vi "Write UDVs.vi"(7 "R/W Case":T4, 8 "error in (no error)":errorcluster, 9 "Input FIFO buffer in":dbl[](array[numeric]), 10 "Input Data in":T1 {"BD Refs"."Data Reference" format="%.0x"}, 11 "UDVs in":T5[](array[typedef]) {"VS ref" format="%.0x"}) -> (0 "error out":errorcluster, 1 "Input FIFO buffer out":dbl[](array[numeric]), 2 "Input Data out":T1 {"BD Refs"."Data Reference" format="%.0x"}, 3 "UDVs out":T5[](array[typedef]) {"VS ref" format="%.0x"})   [LabVIEW 2016, in "Scan Engine Custom Device.lvlib"]
uses:
  Scan Engine Custom Device.lvlib
  Type Defs/UDV Data.ctl
  <vilib>/NI Veristand/Custom Device API/Custom Device Item Ref.ctl
  Type Defs/UDV Data Type.ctl
  Type Defs/FXP Config.ctl
  Type Defs/RW Case.ctl
  Type Defs/Input Data.ctl
  <vilib>/NI Veristand/Custom Device API/Block Data Reference.ctl
  <vilib>/NI Veristand/Custom Device API/Data Reference.ctl
  <vilib>/NI Veristand/Custom Device API/Global Data Refs.vi
  <vilib>/NI Veristand/Custom Device API/Custom Device API.lvlib
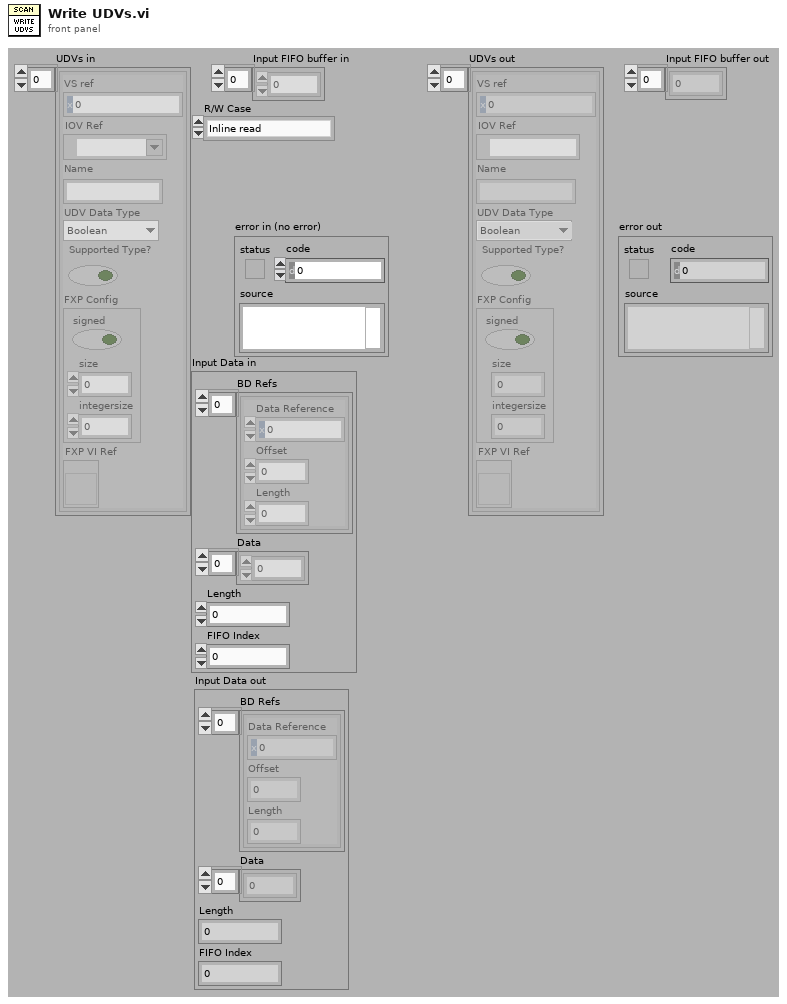
[diagram p1: front panel]
types:
  T1 = typedef "Scan Engine Custom Device.lvlib/Input Data.ctl" = cluster{"BD Refs":T2[], "Data":dbl[], "Length":i32, "FIFO Index":i32}
  T2 = typedef "Custom Device API.lvlib/Block Data Reference.ctl" = cluster{"Data Reference":T3, "Offset":u64, "Length":u64}
  T3 = typedef "Custom Device API.lvlib/Data Reference.ctl" = i32
  T4 = typedef "Scan Engine Custom Device.lvlib/RW Case.ctl" = enum16{"Inline read", "Inline write", "Async - Inline loop read", "Async - Inline loop write", "Async loop (read/write)"}
  T5 = typedef "Scan Engine Custom Device.lvlib/UDV Data.ctl" = cluster{"VS ref":T6, "IOV Ref":refnum<k21>, "Name":string, "UDV Data Type":T7, "Supported Type?":bool, "FXP Config":T8, "FXP VI Ref":refnum<vi>}
  T6 = typedef "Custom Device API.lvlib/Custom Device Item Ref.ctl" = u64
  T7 = typedef "Scan Engine Custom Device.lvlib/UDV Data Type.ctl" = enum16{"Boolean", "Fixed Point", "Int8", "Int16", "Int32", "Int64", "U32 Bit Field", "UInt8", "UInt16", "UInt32", "UInt64", "Other"}
  T8 = typedef "Scan Engine Custom Device.lvlib/FXP Config.ctl" = cluster{"signed":bool, "size":u32, "integersize":i32}
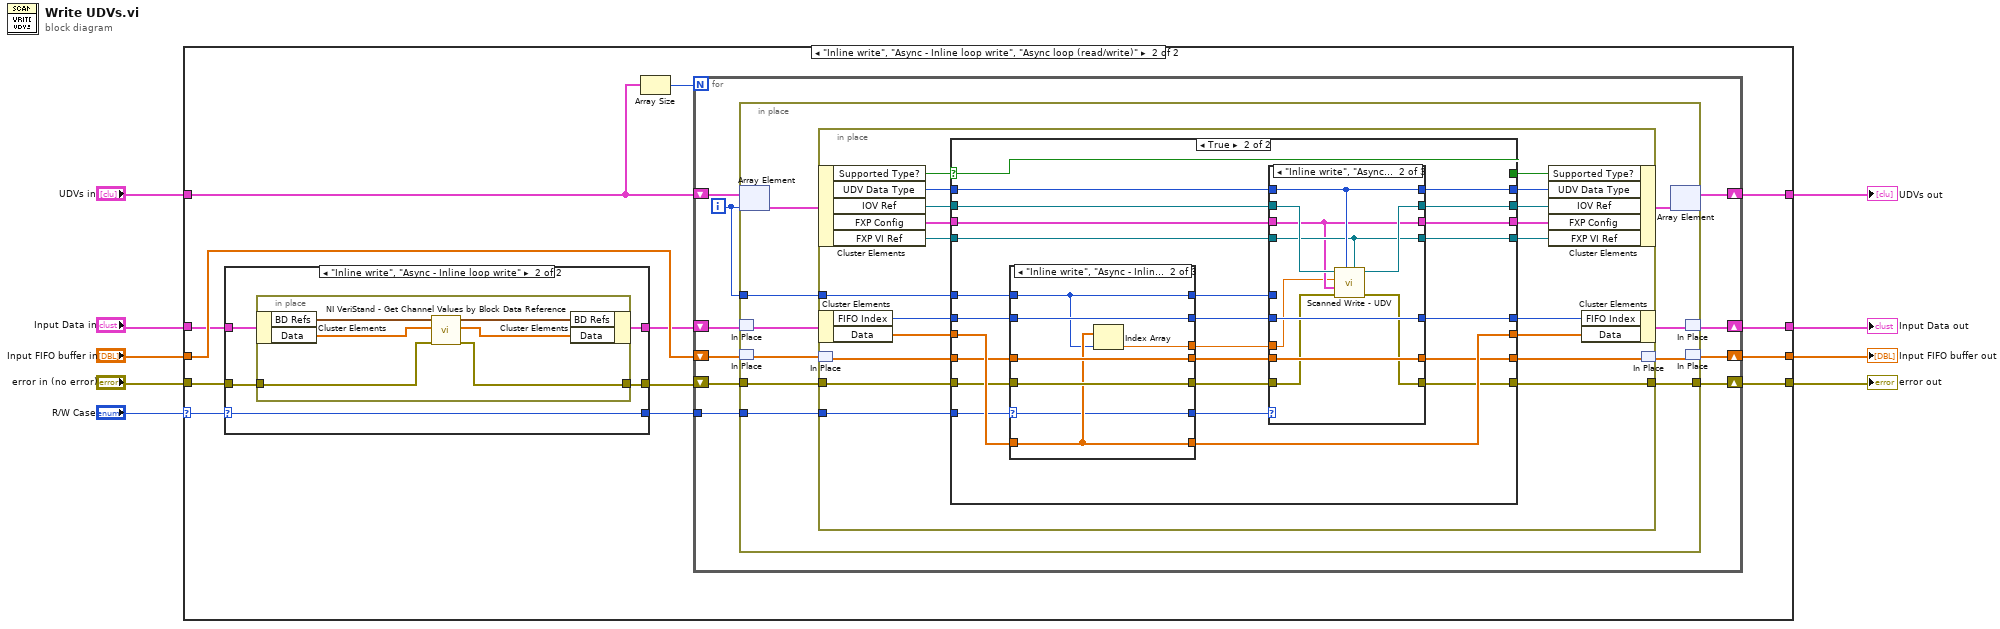
[diagram p0: block diagram]
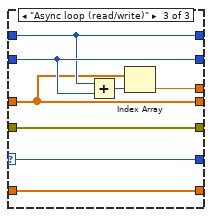
[diagram p6: hidden frame]
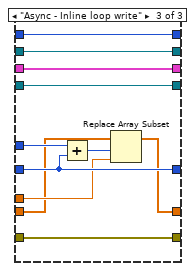
[diagram p8: hidden frame]
diagram:
  n1 = case shown="\"Inline write\", \"Async - Inline loop write\", \"Async loop (read/write)\"" "R/W Case" {
    selector: "R/W Case" -> [_ w21]
    tunnel: [w11 w26] -> w9
    tunnel: "Input FIFO buffer in" -> [w11 w25]
    tunnel: [w12 w15] -> w1
    tunnel: [w13 w24] -> w7
    tunnel: "Input Data in" -> [w12 w19]
    tunnel: "UDVs in" -> [w13 w23]
    tunnel: [w10 w14] -> w5
    tunnel: "error in (no error)" -> [w10 w20]
    frame Default {
    }
    frame "Inline write", "Async - Inline loop write", "Async loop (read/write)" {
      n2 = case shown="\"Inline write\", \"Async - Inline loop write\"" w21 {
        selector: w21 -> [w27 w30]
        tunnel: w19 -> [w28 w34]
        tunnel: w20 -> [w29 w33]
        tunnel: [w29 w32] -> w17
        tunnel: [w28 w31] -> w18
        tunnel: [w27 w30] -> w16
        frame Default {
        }
        frame "Inline write", "Async - Inline loop write" {
          n3 = in-place {
            in-place-border: w33 -> [w36]
            in-place-border: [w35] -> w32
            n4 = in-place-cluster #1(w34) -> ("BD Refs"=w40:T2[], "Data"=w38:dbl[])
            n5 = call <vilib>:"NI VeriStand - Get Channel Values by Block Data Reference.vi"("error in (no error)"=w36, "Values Array in"=w38, "Block Data Ref"=w40) -> ("error out"=w35:errorcluster, "Values Array out"=w37:dbl[], "Block Data Ref dup"=w39:T2[])  [unwired: 6 in]
            n6 = in-place-cluster #1("BD Refs"=w39, "Data"=w37) -> (w31:T1)
          }
        }
      }
      n7 = Array Size(array=w23) -> (size(s)=w22:i32)
      n8 = for {
        N: w22 -> [_]
        shift-right: [w49] -> w24
        shift-left: w23 -> [w50]
        shift-right: [w41] -> w15
        shift-left: w18 -> [w44]
        shift-right: [w47] -> w26
        shift-left: w25 -> [w48]
        shift-right: [w45] -> w14
        shift-left: w17 -> [w46]
        tunnel: w16 -> [w43]
        i -> [w42]
        n9 = in-place {
          in-place-border: w46 -> [w57]
          in-place-border: [w51] -> w45
          in-place-border: w43 -> [w56]
          in-place-border: w42 -> [w55]
          n10 = in-place-array #2(w50, w42) -> (w60:T5)
          n11 = in-place-match #3(w44) -> (w59:T1)
          n12 = in-place-match #4(w48) -> (w58:dbl[])
          n13 = in-place {
            in-place-border: w57 -> [w71]
            in-place-border: w56 -> [w61]
            in-place-border: w55 -> [w72]
            in-place-border: [w65] -> w51
            n14 = in-place-cluster #5(w60) -> ("Supported Type?"=w80:bool, "UDV Data Type"=w75:T7, "IOV Ref"=w74:refnum<k21>, "FXP Config"=w79:T8, "FXP VI Ref"=w78:refnum<vi>)
            n15 = in-place-cluster #6(w59) -> ("FIFO Index"=w77:i32, "Data"=w76:dbl[])
            n16 = in-place-match #7(w58) -> (w73:dbl[])
            n17 = case shown="True" w80 {
              selector: w80 -> [w88 w110]
              tunnel: w79 -> [w85 w112]
              tunnel: w78 -> [w84 w111]
              tunnel: w77 -> [w83 w100]
              tunnel: w76 -> [w82 w105]
              tunnel: w75 -> [w87 w114]
              tunnel: w74 -> [w86 w113]
              tunnel: w73 -> [w81 w99]
              tunnel: w72 -> [_ w101]
              tunnel: w71 -> [w89 w98]
              tunnel: [w88 w110] -> w70
              tunnel: [w87 w109] -> w69
              tunnel: [w86 w108] -> w68
              tunnel: [w85 w107] -> w67
              tunnel: [w84 w106] -> w66
              tunnel: [w89 w90] -> w65
              tunnel: [w83 w92] -> w64
              tunnel: [w82 w104] -> w63
              tunnel: [w81 w91] -> w62
              tunnel: w61 -> [_ w103]
              frame False {
              }
              frame True {
                n18 = case shown="\"Inline write\", \"Async - Inline loop write\"" w103 {
                  selector: w103 -> [w117 w121 w128]
                  tunnel: w101 -> [w115 w122 w130]
                  tunnel: w100 -> [w120 w125 w133]
                  tunnel: w99 -> [w118 w126 w129]
                  tunnel: w98 -> [w116 w127 w135]
                  tunnel: w105 -> [w119 w123 w134]
                  tunnel: [w120 w125 w133] -> w95
                  tunnel: [w119 w123 w134] -> w104
                  tunnel: [w116 w127 w135] -> w97
                  tunnel: [w118 w126 w129] -> w94
                  tunnel: [w117 w121 w128] -> w102
                  tunnel: [_ w124 w131] -> w93
                  tunnel: [w115 w122 w130] -> w96
                  frame Default {
                  }
                  frame "Inline write", "Async - Inline loop write" {
                    n19 = Index Array(array=w123, index=w122) -> (element=w124:dbl)
                  }
                  frame "Async loop (read/write)" {
                    n20 = Add(x=w130, y=w133) -> (x+y=w132:i32)
                    n21 = Index Array(array=w129, index=w132) -> (element=w131:dbl)
                  }
                }
                n22 = case shown="\"Inline write\", \"Async loop (read/write)\"" w102 {
                  tunnel: w114 -> [w136 w148 w161]
                  tunnel: w113 -> [w137 w150 w153]
                  tunnel: w112 -> [w138 w146 w163]
                  tunnel: w111 -> [w139 w147 w162]
                  tunnel: w95 -> [w140 w151 w158]
                  tunnel: w94 -> [w141 w152 w155]
                  tunnel: [w141 w152 w154] -> w91
                  tunnel: w96 -> [_ _ w159]
                  tunnel: [w140 w151 w158] -> w92
                  tunnel: [w137 w149 w153] -> w108
                  tunnel: [w136 w148 w161] -> w109
                  tunnel: [w138 w146 w163] -> w107
                  tunnel: [w139 w147 w162] -> w106
                  tunnel: w97 -> [w142 w144 w160]
                  tunnel: [w142 w143 w160] -> w90
                  tunnel: w93 -> [_ w145 w156]
                  frame Default {
                  }
                  frame "Inline write", "Async loop (read/write)" {
                    n23 = call "Scanned Write - UDV.vi"("FXP VI Ref"=w147, "UDV Data Type"=w148, "error in (no error)"=w144, "FXP Config"=w146, "data in"=w145, "IOV ref in"=w150) -> ("error out"=w143:errorcluster, "IOV ref out"=w149:refnum<k21>)  [unwired: 4 in]
                  }
                  frame "Async - Inline loop write" {
                    n24 = Add(x=w159, y=w158) -> (x+y=w157:i32)
                    n25 = Replace Array Subset(array=w155, new element=w156, index=w157) -> (w154:dbl[])
                  }
                }
              }
            }
            n26 = in-place-cluster #5("Supported Type?"=w70, "UDV Data Type"=w69, "IOV Ref"=w68, "FXP Config"=w67, "FXP VI Ref"=w66) -> (w54:T5)
            n27 = in-place-cluster #6("FIFO Index"=w64, "Data"=w63) -> (w53:T1)
            n28 = in-place-match #7(w62) -> (w52:dbl[])
          }
          n29 = in-place-array #2(w54) -> (w49:T5[])  [unwired: 1 out]
          n30 = in-place-match #3(w53) -> (w41:T1)
          n31 = in-place-match #4(w52) -> (w47:dbl[])
        }
      }
    }
  }
  "Input FIFO buffer out" <- w9
  "UDVs out" <- w7
  "error out" <- w5
  "Input Data out" <- w1
